vi "Move Stage.vi"(0 ".NET Refnum in":refnum<k24>, 5 "New Position":dbl, 11 "error in (no error)":errorcluster) -> (4 ".NET Refnum out":refnum<k24>, 15 "error out":errorcluster)   [LabVIEW 2013, in "ThorlabsLTS.lvclass"]
uses:
  ThorlabsLTS.lvclass
  C:/GEECS/Developers Version/source/Device Driver/ThorLabsLTS/Thorlabs.MotionControl.IntegratedStepperMotorsCLI.dll
  Thorlabs.MotionControl.IntegratedStepperMotorsCLI.dll
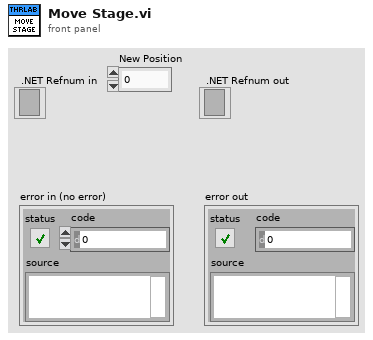
[diagram p1: front panel]
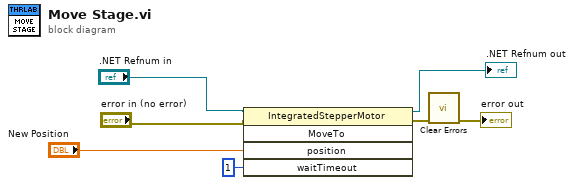
[diagram p0: block diagram]
diagram:
  n1 = invoke class="IntegratedStepperMotor" method="MoveTo"(reference=".NET Refnum in", error in="error in (no error)", "position"="New Position", "waitTimeout"=1) -> (reference out=→".NET Refnum out":refnum<k24>, error out=w4:errorcluster)  [unwired: 1 in, 3 out]
  n2 = call <vilib>:"Clear Errors.vi"("error in (no error)"=w4) -> ("error out"=→"error out":errorcluster)  [unwired: 6 in]
